vi "FileIO-Read Anything.vi"(6 "Prompt?":bool, 7 "Type of Anything":variant, 8 "error in (no error)":errorcluster, 9 "Section Name":string, 11 "Settings file":path) -> (0 "error out":errorcluster, 2 "Anything":variant, 3 "Path out":path, 4 "Read?":bool)   [LabVIEW 2020]
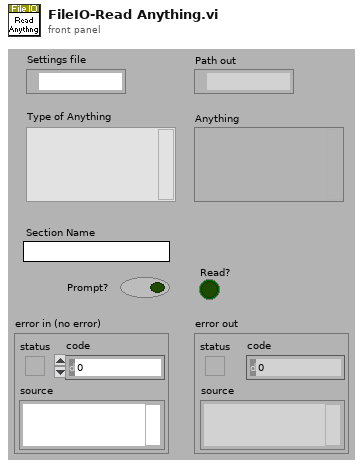
[diagram p1: front panel]
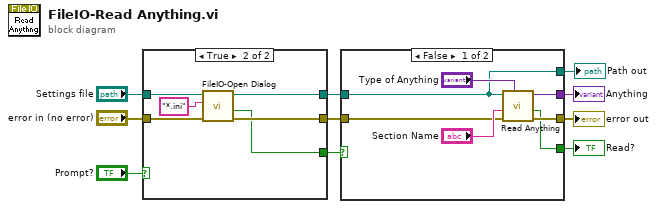
[diagram p0: block diagram]
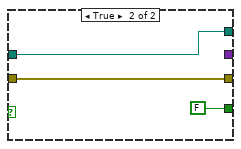
[diagram p2: hidden frame]
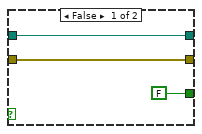
[diagram p3: hidden frame]
diagram:
  n1 = case shown="True" "Prompt?" {
    tunnel: "Settings file" -> [w13 w19]
    tunnel: "error in (no error)" -> [w12 w17]
    tunnel: [w12 w16] -> w6
    tunnel: [w13 w15] -> w5
    tunnel: [FALSE ("cancelled") w14] -> w7
    frame False {
    }
    frame True {
      n2 = call "FileIO-Open Dialog.vi"("error in"=w17, "pattern (all files)"="*.ini", "Start path"=w19) -> ("error out"=w16:errorcluster, "cancelled"=w14:bool, "selected path"=w15:path)  [unwired: 6 in]
    }
  }
  n3 = case shown="False" w7 {
    tunnel: w6 -> [w25 w29]
    tunnel: w5 -> [w21 w27]
    tunnel: [w24 _] -> w2
    tunnel: [w23 w29] -> w4
    tunnel: [w20 FALSE] -> w3
    tunnel: [w21 w27] -> w1
    frame False {
      n4 = call "Read Anything.vi"("Type of Anything"="Type of Anything", "Error In"=w25, "Section Name (Name of \"Type of Anything\")"="Section Name", "Path (dialog)"=w21) -> ("Error Out"=w23:errorcluster, "Found?"=w20:bool, "Anything"=w24:variant)  [unwired: 5 in]
    }
    frame True {
    }
  }
  "error out" <- w4
  "Read?" <- w3
  "Path out" <- w1
  "Anything" <- w2
